vi "GetSubPanState.vi"(8 "ErrorIn(No Error)":errorcluster caption="entrée d'erreur (pas d'erreur)", 11 "référence":refnum<vi>) -> (0 "sortie d'erreur":errorcluster, 1 "FA_Closed":bool, 2 "Vi_Running":bool, 3 "Ref_Out":refnum<vi>)   [LabVIEW 2010]
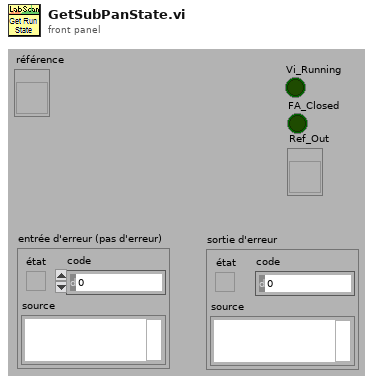
[diagram p1: front panel]
types:
  T1 = enum32{"Invalid", "Standard", "Closed", "Hidden", "Minimized", "Maximized"}
  T2 = enum32{"Bad", "Idle", "Run top level", "Running"}
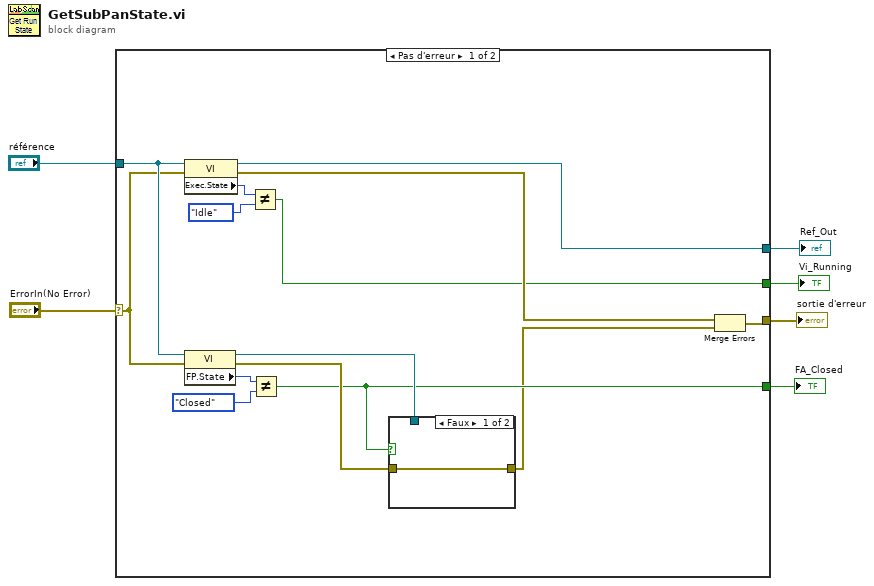
[diagram p0: block diagram]
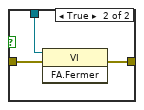
[diagram p2: hidden frame]
diagram:
  n1 = case shown="Pas d'erreur" "ErrorIn(No Error)" {
    selector: "ErrorIn(No Error)" -> [w12 w26]
    tunnel: [w10 w26] -> w5
    tunnel: [w14 _] -> w4
    tunnel: "référence" -> [w13 w25]
    tunnel: [w11 w25] -> w2
    tunnel: [w7 _] -> w1
    frame No Error {
      n2 = property class="VI"(reference=w13, error in=w12) -> (reference out=w11:refnum<vi>, error out=w8:errorcluster, "Exec.State"=w19:T2)
      n3 = property class="VI"(reference=w13, error in=w12) -> (reference out=w15:refnum<vi>, error out=w16:errorcluster, "FP.State"=w18:T1)
      n4 = Not Equal?(x=w19, y=T2."Idle" ("Exécution : état")) -> (x != y?=w7:bool)
      n5 = Not Equal?(x=w18, y=T1."Closed" ("Fenêtre face-avant : état")) -> (x != y?=w14:bool)
      n6 = case shown="Faux" w14 {
        tunnel: w15 -> [_ w24]
        tunnel: w16 -> [w21 w23]
        tunnel: [w21 w22] -> w9
        frame False {
        }
        frame True {
          n7 = invoke class="VI" method="FA.Fermer"(reference=w24, error in=w23) -> (error out=w22:errorcluster)  [unwired: 1 in, 2 out]
        }
      }
      n8 = Merge Errors(w8, w9) -> (w10:errorcluster)
    }
    frame Error {
    }
  }
  "sortie d'erreur" <- w5
  "FA_Closed" <- w4
  "Ref_Out" <- w2
  "Vi_Running" <- w1
